vi "itc4000.vi"(9 "Temperatura":dbl min=-10.00001 max=69.99999, 10 "Corriente":dbl min=0.0 max=0.001 step=1e-05) -> (0 "Temperatura sal":dbl, 1 "Corriente sal":dbl, 2 "Power (0)":dbl)   [LabVIEW 2016]
panel:
  out "error out":errorcluster
  in  "Error In":errorcluster
  out "TEC Current":dbl
  out "TEC Voltage":dbl
  out "TEC Power":dbl
  in  "stop":bool
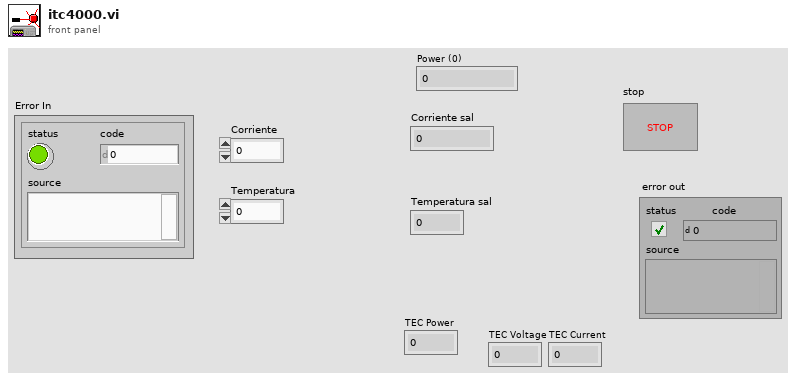
[diagram p1: front panel]
types:
  T1 = enum16{"inicio", "configurarGUI", "VALORESDEFAULT", "valordef2", "limites", "delay", "medir", "cerrar"}
  T2 = enum8{"Enabled", "Disabled", "Disabled and Grayed Out"}
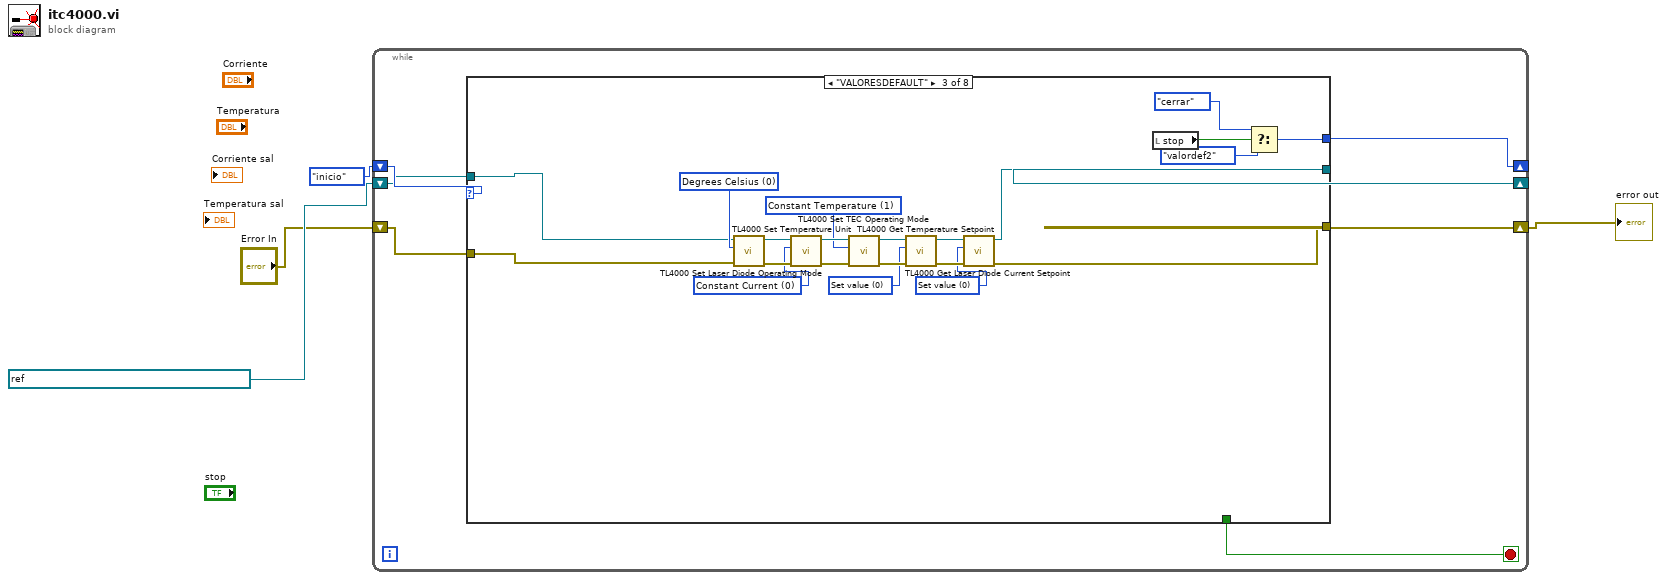
[diagram p0: block diagram]
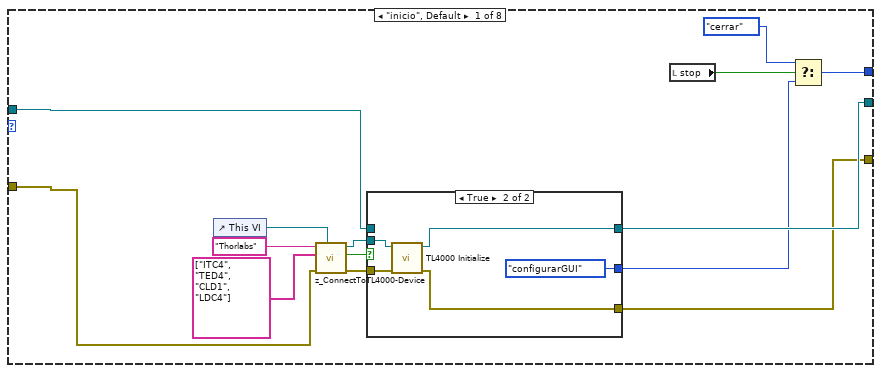
[diagram p2: hidden frame]
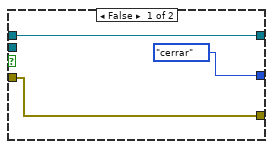
[diagram p3: hidden frame]
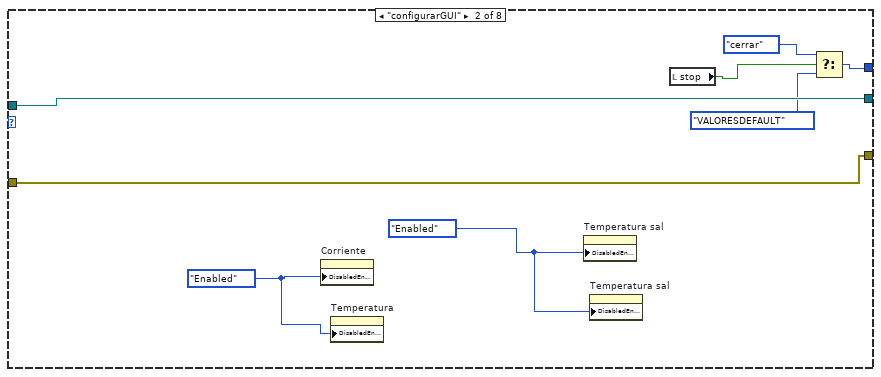
[diagram p4: hidden frame]
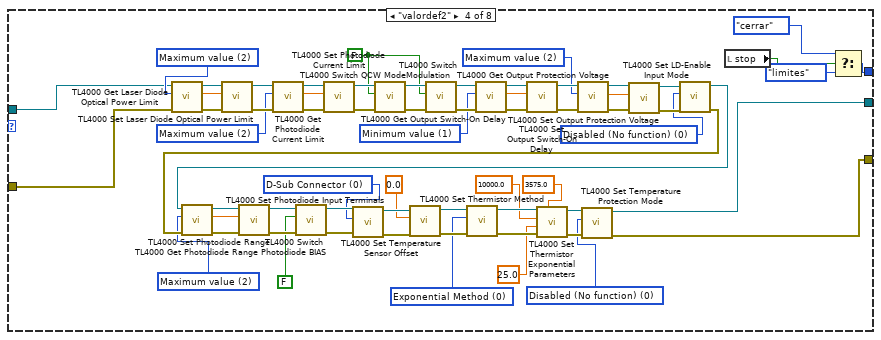
[diagram p5: hidden frame]
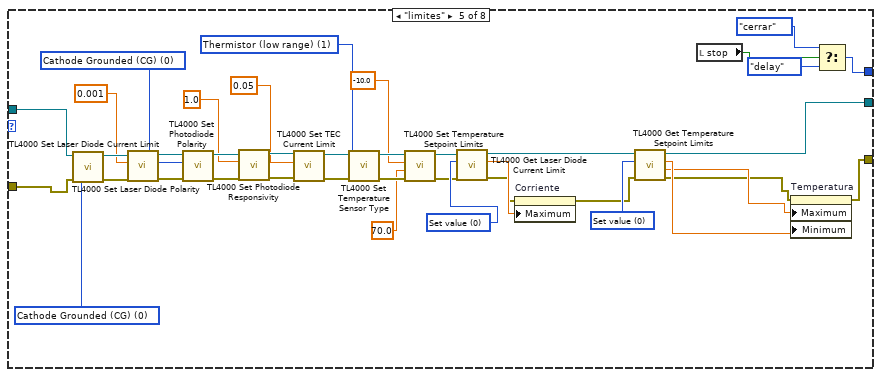
[diagram p6: hidden frame]
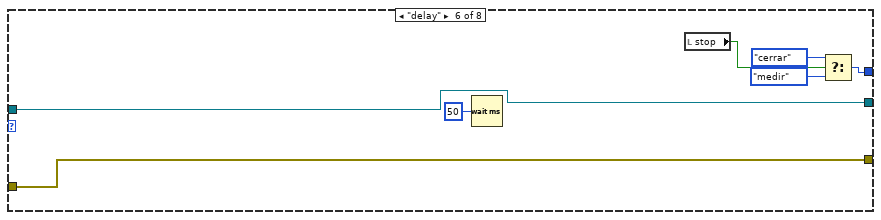
[diagram p7: hidden frame]
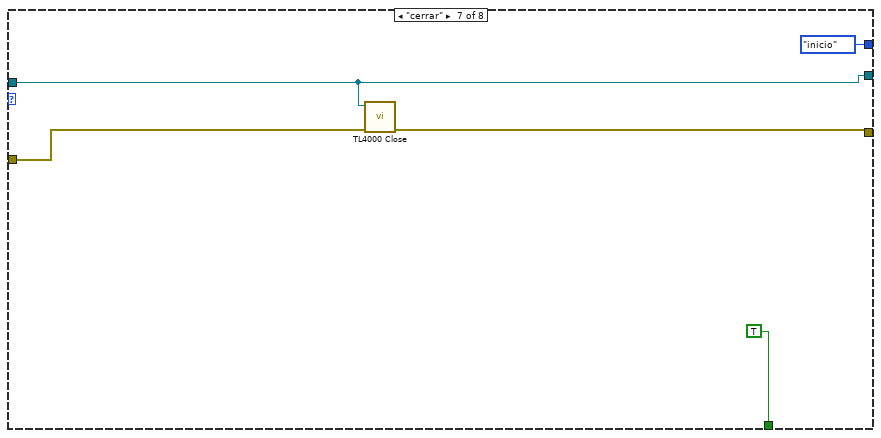
[diagram p8: hidden frame]
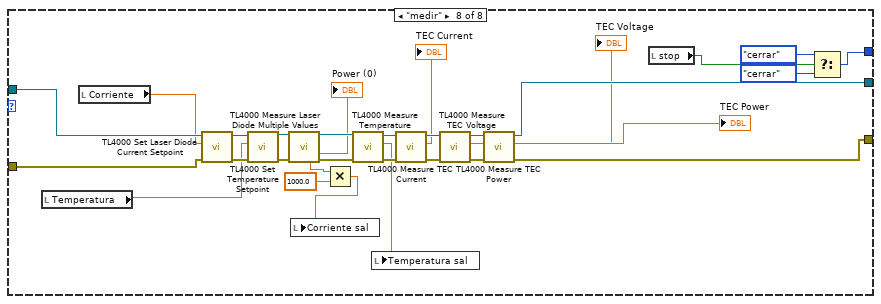
[diagram p9: hidden frame]
diagram:
  n1 = while {
    shift-right: [w6] -> _
    shift-left: T1."inicio" -> [w11]
    shift-right: [w10] -> _
    shift-left: refnum<visa-resource-name> "USB0::0x1313::0x804A::M00534841::INSTR" ("resource name") -> [w8]
    shift-right: [w9] -> w1
    shift-left: "Error In" -> [w7]
    stop <- w5 stop-if-true
    n2 = case shown="\"VALORESDEFAULT\"" w11 {
      tunnel: [w16 w41 w49 w70 w161 w171 w177 w191] -> w10
      tunnel: [w13 w40 w48 w69 w155 w170 w175 w190] -> w9
      tunnel: w8 -> [w15 w41 w47 w68 w135 w171 w177 w193]
      tunnel: w7 -> [w14 w40 w46 w67 w136 w170 w176 w192]
      tunnel: [w24 w34 w42 w64 w151 w168 T1."inicio" ("f") w179] -> w6
      tunnel: [_ _ _ _ _ _ TRUE _] -> w5
      frame "inicio", Default {
        n3 = control-ref of="This VI"() -> (w21:refnum<vi>)
        n4 = call <instrlib>:"z_ConnectToTL4000-Device.vi"("VI reference"=w21, "error in"=w14, "Models"=string[] ["ITC4", "TED4", "CLD1", "LDC4"], "Manufacturer"="Thorlabs") -> ("error out"=w18:errorcluster, "FoundUSB"=w20:bool, "USB Ref"=w19:refnum<visa-resource-name>)  [unwired: 5 in]
        n5 = case shown="True" w20 {
          tunnel: w19 -> [_ w31]
          tunnel: w18 -> [w27 w33]
          tunnel: [T1."cerrar" T1."configurarGUI"] -> w12
          tunnel: [w27 w32] -> w13
          tunnel: [w28 w30] -> w16
          tunnel: w15 -> [w28 _]
          frame False {
          }
          frame True {
            n6 = call <instrlib>:"TL4000 Initialize.vi"("error in (no error)"=w33, "resource name"=w31) -> ("error out"=w32:errorcluster, "instrument handle out"=w30:refnum<visa-resource-name>)  [unwired: 8 in]
          }
        }
        n7 = local read "stop"() -> (w25:bool)
        n8 = Select(t=T1."cerrar", s=w25, f=w12) -> (s? t:f=w24:T1)
      }
      frame "configurarGUI" {
        w38 = T2."Enabled" ("Disabled")
        w39 = T2."Enabled" ("Disabled")
        n9 = property on="Corriente" class="DigNum (strict)"("DisabledEnum"=w39) -> ()  [unwired: 2 in, 2 out]
        n10 = property on="Temperatura" class="DigNum (strict)"("DisabledEnum"=w39) -> ()  [unwired: 2 in, 2 out]
        n11 = property on="Temperatura sal" class="DigNum (strict)"("DisabledEnum"=w38) -> ()  [unwired: 2 in, 2 out]
        n12 = property on="Temperatura sal" class="DigNum (strict)"("DisabledEnum"=w38) -> ()  [unwired: 2 in, 2 out]
        n13 = local read "stop"() -> (w36:bool)
        n14 = Select(t=T1."cerrar", s=w36, f=T1."VALORESDEFAULT") -> (s? t:f=w34:T1)
      }
      frame "VALORESDEFAULT" {
        w50 = i16 0 items=["Set value", "Minimum value", "Maximum value"] ("Attribute (Set value)")
        w51 = i16 0 items=["Set value", "Minimum value", "Maximum value"] ("Attribute (Set value)")
        w52 = i16 1 items=["Constant Temperature"=1, "Current Source"=0] ("TEC Operating Mode (Constant Temperature)")
        w53 = i16 0 items=["Constant Current", "Constant Power"] ("Laser Diode Operating Mode (Constant Current)")
        w54 = i16 0 items=["Degrees Celsius", "Kelvin", "Degrees Fahrenheit"] ("Temperature Unit (Degrees Celsius)")
        n15 = call <instrlib>:"TL4000 Set Temperature Unit.vi"("error in (no error)"=w46, "Temperature Unit (Degrees Celsius)"=w54, "instrument handle"=w47) -> ("error out"=w62:errorcluster, "instrument handle out"=w58:refnum<visa-resource-name>)  [unwired: 7 in]
        n16 = call <instrlib>:"TL4000 Set Laser Diode Operating Mode.vi"("error in (no error)"=w62, "Laser Diode Operating Mode (Constant Current)"=w53, "instrument handle"=w58) -> ("error out"=w61:errorcluster, "instrument handle out"=w57:refnum<visa-resource-name>)  [unwired: 7 in]
        n17 = call <instrlib>:"TL4000 Set TEC Operating Mode.vi"("error in (no error)"=w61, "TEC Operating Mode (Constant Temperature)"=w52, "instrument handle"=w57) -> ("error out"=w60:errorcluster, "instrument handle out"=w56:refnum<visa-resource-name>)  [unwired: 7 in]
        n18 = call <instrlib>:"TL4000 Get Laser Diode Current Setpoint.vi"("error in (no error)"=w60, "Attribute (Set value)"=w51, "instrument handle"=w56) -> ("error out"=w59:errorcluster, "instrument handle out"=w55:refnum<visa-resource-name>)  [unwired: 6 in, 1 out]
        n19 = call <instrlib>:"TL4000 Get Temperature Setpoint.vi"("error in (no error)"=w59, "Attribute (Set value)"=w50, "instrument handle"=w55) -> ("error out"=w48:errorcluster, "instrument handle out"=w49:refnum<visa-resource-name>)  [unwired: 6 in, 1 out]
        n20 = local read "stop"() -> (w44:bool)
        n21 = Select(t=T1."cerrar", s=w44, f=T1."valordef2") -> (s? t:f=w42:T1)
      }
      frame "valordef2" {
        w71 = i16 0 items=["Disabled (No function)", "Output Enable", "Output Protection"] ("Mode (Disabled (No function))")
        w72 = i16 0 items=["Exponential Method", "Method from Steinhart-Hart"] ("Method (Exponential Method)")
        w74 = i16 0 items=["D-Sub Connector", "Rear Panel BNC"] ("Terminals (D-Sub Connector)")
        w76 = i16 2 items=["Set value", "Minimum value", "Maximum value"] ("Attribute (Set value)")
        w78 = i16 0 items=["Disabled (No function)", "Output Enable", "Output Protection"] ("Mode (Disabled (No function))")
        w80 = i16 2 items=["Set value", "Minimum value", "Maximum value", "Default value"] ("Attribute (Set value)")
        w82 = i16 1 items=["Set value", "Minimum value", "Maximum value", "Default value"] ("Attribute (Set value)")
        w83 = FALSE ("QCW Mode (Off)")
        w85 = i16 2 items=["Set value", "Minimum value", "Maximum value"] ("Attribute (Set value)")
        w87 = i16 2 items=["Set value", "Minimum value", "Maximum value"] ("Attribute (Set value)")
        n22 = call <instrlib>:"TL4000 Get Laser Diode Optical Power Limit.vi"("error in (no error)"=w67, "Attribute (Set value)"=w87, "instrument handle"=w68) -> ("error out"=w125:errorcluster, "Optical Power Limit"=w86:dbl, "instrument handle out"=w126:refnum<visa-resource-name>)  [unwired: 6 in]
        n23 = call <instrlib>:"TL4000 Set Laser Diode Optical Power Limit.vi"("error in (no error)"=w125, "Optical Power Limit (0.0)"=w86, "instrument handle"=w126) -> ("error out"=w123:errorcluster, "instrument handle out"=w124:refnum<visa-resource-name>)  [unwired: 7 in]
        n24 = call <instrlib>:"TL4000 Get Photodiode Current Limit.vi"("error in (no error)"=w123, "Attribute (Set value)"=w85, "instrument handle"=w124) -> ("error out"=w121:errorcluster, "Photodiode Current Limit"=w84:dbl, "instrument handle out"=w122:refnum<visa-resource-name>)  [unwired: 6 in]
        n25 = call <instrlib>:"TL4000 Set Photodiode Current Limit.vi"("error in (no error)"=w121, "Photodiode Current Limit (0.0)"=w84, "instrument handle"=w122) -> ("error out"=w119:errorcluster, "instrument handle out"=w120:refnum<visa-resource-name>)  [unwired: 7 in]
        n26 = call <instrlib>:"TL4000 Switch QCW Mode.vi"("error in (no error)"=w119, "QCW Mode (Off)"=w83, "instrument handle"=w120) -> ("error out"=w117:errorcluster, "instrument handle out"=w118:refnum<visa-resource-name>)  [unwired: 7 in]
        n27 = call <instrlib>:"TL4000 Switch Modulation.vi"("error in (no error)"=w117, "Modulation State (Off)"=w83, "instrument handle"=w118) -> ("error out"=w115:errorcluster, "instrument handle out"=w116:refnum<visa-resource-name>)  [unwired: 7 in]
        n28 = call <instrlib>:"TL4000 Get Output Switch-On Delay.vi"("error in (no error)"=w115, "Attribute (Set value)"=w82, "instrument handle"=w116) -> ("error out"=w113:errorcluster, "Delay"=w81:dbl, "instrument handle out"=w114:refnum<visa-resource-name>)  [unwired: 6 in]
        n29 = call <instrlib>:"TL4000 Set Output Switch-On Delay.vi"("error in (no error)"=w113, "Delay (1.0)"=w81, "instrument handle"=w114) -> ("error out"=w111:errorcluster, "instrument handle out"=w112:refnum<visa-resource-name>)  [unwired: 7 in]
        n30 = call <instrlib>:"TL4000 Get Output Protection Voltage.vi"("error in (no error)"=w111, "Attribute (Set value)"=w80, "instrument handle"=w112) -> ("error out"=w109:errorcluster, "Voltage"=w79:dbl, "instrument handle out"=w110:refnum<visa-resource-name>)  [unwired: 6 in]
        n31 = call <instrlib>:"TL4000 Set Output Protection Voltage.vi"("error in (no error)"=w109, "Voltage (5.0)"=w79, "instrument handle"=w110) -> ("error out"=w108:errorcluster, "instrument handle out"=w107:refnum<visa-resource-name>)  [unwired: 7 in]
        n32 = call <instrlib>:"TL4000 Set LD-Enable Input Mode.vi"("error in (no error)"=w108, "Mode (Disabled (No function))"=w78, "instrument handle"=w107) -> ("error out"=w105:errorcluster, "instrument handle out"=w106:refnum<visa-resource-name>)  [unwired: 7 in]
        n33 = call <instrlib>:"TL4000 Get Photodiode Range.vi"("error in (no error)"=w105, "Attribute (Set value)"=w76, "instrument handle"=w106) -> ("error out"=w103:errorcluster, "Range"=w77:dbl, "instrument handle out"=w104:refnum<visa-resource-name>)  [unwired: 6 in]
        n34 = call <instrlib>:"TL4000 Set Photodiode Range.vi"("error in (no error)"=w103, "Range (0.001)"=w77, "instrument handle"=w104) -> ("error out"=w101:errorcluster, "instrument handle out"=w102:refnum<visa-resource-name>)  [unwired: 7 in]
        n35 = call <instrlib>:"TL4000 Switch Photodiode BIAS.vi"("error in (no error)"=w101, "BIAS State (Off)"=FALSE, "instrument handle"=w102) -> ("error out"=w99:errorcluster, "instrument handle out"=w100:refnum<visa-resource-name>)  [unwired: 7 in]
        n36 = call <instrlib>:"TL4000 Set Photodiode Input Terminals.vi"("error in (no error)"=w99, "Terminals (D-Sub Connector)"=w74, "instrument handle"=w100) -> ("error out"=w97:errorcluster, "instrument handle out"=w98:refnum<visa-resource-name>)  [unwired: 7 in]
        n37 = call <instrlib>:"TL4000 Set Temperature Sensor Offset.vi"("error in (no error)"=w97, "Temperature Offset (0.0)"=0.0, "instrument handle"=w98) -> ("error out"=w95:errorcluster, "instrument handle out"=w96:refnum<visa-resource-name>)  [unwired: 7 in]
        n38 = call <instrlib>:"TL4000 Set Thermistor Method.vi"("error in (no error)"=w95, "Method (Exponential Method)"=w72, "instrument handle"=w96) -> ("error out"=w91:errorcluster, "instrument handle out"=w92:refnum<visa-resource-name>)  [unwired: 7 in]
        n39 = call <instrlib>:"TL4000 Set Thermistor Exponential Parameters.vi"("Beta value (3575.0)"=3575.0, "error in (no error)"=w91, "T0 value (25.0)"=25.0, "R0 value (10.0E3)"=10000.0, "instrument handle"=w92) -> ("error out"=w93:errorcluster, "instrument handle out"=w94:refnum<visa-resource-name>)  [unwired: 5 in]
        n40 = call <instrlib>:"TL4000 Set Temperature Protection Mode.vi"("error in (no error)"=w93, "Mode (Disabled (No function))"=w71, "instrument handle"=w94) -> ("error out"=w69:errorcluster, "instrument handle out"=w70:refnum<visa-resource-name>)  [unwired: 7 in]
        n41 = local read "stop"() -> (w65:bool)
        n42 = Select(t=T1."cerrar", s=w65, f=T1."limites") -> (s? t:f=w64:T1)
      }
      frame "limites" {
        w129 = i16 1 items=["AD590", "Thermistor (low range)", "Thermistor (high range)", "PT100", "PT1000", "LM35", "LM335"] ("Sensor (AD590)")
        w132 = i16 0 items=["Cathode Grounded (CG)", "Anode Grounded (AG)"] ("Polarity (Cathode Grounded (CG))")
        w134 = i16 0 items=["Cathode Grounded (CG)", "Anode Grounded (AG)"] ("Polarity (Cathode Grounded (CG))")
        w165 = i16 0 items=["Set value", "Minimum value", "Maximum value"] ("Attribute (Set value)")
        w164 = i16 0 items=["Set value", "Minimum value", "Maximum value"] ("Attribute (Set value)")
        n43 = call <instrlib>:"TL4000 Set Laser Diode Polarity.vi"("error in (no error)"=w136, "Polarity (Cathode Grounded (CG))"=w134, "instrument handle"=w135) -> ("error out"=w149:errorcluster, "instrument handle out"=w150:refnum<visa-resource-name>)  [unwired: 7 in]
        n44 = call <instrlib>:"TL4000 Set Laser Diode Current Limit.vi"("error in (no error)"=w149, "Laser Diode Current Limit (0.0)"=0.001, "instrument handle"=w150) -> ("error out"=w147:errorcluster, "instrument handle out"=w148:refnum<visa-resource-name>)  [unwired: 7 in]
        n45 = call <instrlib>:"TL4000 Set Photodiode Polarity.vi"("error in (no error)"=w147, "Polarity (Cathode Grounded (CG))"=w132, "instrument handle"=w148) -> ("error out"=w145:errorcluster, "instrument handle out"=w146:refnum<visa-resource-name>)  [unwired: 7 in]
        n46 = call <instrlib>:"TL4000 Set Photodiode Responsivity.vi"("error in (no error)"=w145, "Responsivity (1.0)"=1.0, "instrument handle"=w146) -> ("error out"=w143:errorcluster, "instrument handle out"=w144:refnum<visa-resource-name>)  [unwired: 7 in]
        n47 = call <instrlib>:"TL4000 Set TEC Current Limit.vi"("error in (no error)"=w143, "TEC Current Limit (1.0)"=0.05, "instrument handle"=w144) -> ("error out"=w141:errorcluster, "instrument handle out"=w142:refnum<visa-resource-name>)  [unwired: 7 in]
        n48 = call <instrlib>:"TL4000 Set Temperature Sensor Type.vi"("error in (no error)"=w141, "Sensor (AD590)"=w129, "instrument handle"=w142) -> ("error out"=w139:errorcluster, "instrument handle out"=w140:refnum<visa-resource-name>)  [unwired: 7 in]
        n49 = call <instrlib>:"TL4000 Set Temperature Setpoint Limits.vi"("error in (no error)"=w139, "Setpoint High Limit (50.0)"=70.0, "Setpoint Low Limit (0.0)"=-10.0, "instrument handle"=w140) -> ("error out"=w137:errorcluster, "instrument handle out"=w138:refnum<visa-resource-name>)  [unwired: 6 in]
        n50 = call <instrlib>:"TL4000 Get Laser Diode Current Limit.vi"("error in (no error)"=w137, "Attribute (Set value)"=w164, "instrument handle"=w138) -> ("error out"=w157:errorcluster, "Laser Diode Current Limit"=w162:dbl, "instrument handle out"=w163:refnum<visa-resource-name>)  [unwired: 6 in]
        n51 = property on="Corriente" class="DigNum (strict)"(error in=w157, "Maximum"=w162) -> (error out=w156:errorcluster)  [unwired: 1 in, 1 out]
        n52 = call <instrlib>:"TL4000 Get Temperature Setpoint Limits.vi"("error in (no error)"=w156, "Attribute (Set value)"=w165, "instrument handle"=w163) -> ("error out"=w158:errorcluster, "Setpoint High Limit"=w159:dbl, "Setpoint Low Limit"=w160:dbl, "instrument handle out"=w161:refnum<visa-resource-name>)  [unwired: 5 in]
        n53 = local read "stop"() -> (w153:bool)
        n54 = property on="Temperatura" class="DigNum (strict)"(error in=w158, "Maximum"=w159, "Minimum"=w160) -> (error out=w155:errorcluster)  [unwired: 1 in, 1 out]
        n55 = Select(t=T1."cerrar", s=w153, f=T1."delay") -> (s? t:f=w151:T1)
      }
      frame "delay" {
        n56 = Wait (ms)(milliseconds to wait=u32 50) -> ()  [unwired: 1 out]
        n57 = local read "stop"() -> (w167:bool)
        n58 = Select(t=T1."cerrar", s=w167, f=T1."medir") -> (s? t:f=w168:T1)
      }
      frame "cerrar" {
        n59 = call <instrlib>:"TL4000 Close.vi"("error in (no error)"=w176, "instrument handle"=w177) -> ("error out"=w175:errorcluster)  [unwired: 9 in]
      }
      frame "medir" {
        n60 = local read "Temperatura"() -> (w183:dbl)
        n61 = local read "Corriente"() -> (w178:dbl)
        n62 = call <instrlib>:"TL4000 Set Laser Diode Current Setpoint.vi"("error in (no error)"=w192, "Laser Diode Current Setpoint (0.0)"=w178, "instrument handle"=w193) -> ("error out"=w194:errorcluster, "instrument handle out"=w195:refnum<visa-resource-name>)  [unwired: 7 in]
        n63 = call <instrlib>:"TL4000 Set Temperature Setpoint.vi"("error in (no error)"=w194, "Temperature Setpoint (25.0)"=w183, "instrument handle"=w195) -> ("error out"=w202:errorcluster, "instrument handle out"=w203:refnum<visa-resource-name>)  [unwired: 7 in]
        n64 = call <instrlib>:"TL4000 Measure Laser Diode Multiple Values.vi"("instrument handle"=w203, "error in (no error)"=w202) -> ("instrument handle out"=w200:refnum<visa-resource-name>, "Power (0)"=→"Power (0)":dbl, "Photodiode Current (0)"=w197:dbl, "error out"=w201:errorcluster)  [unwired: 5 in, 5 out]
        n65 = Multiply(x=w197, y=1000.0) -> (x*y=w184:dbl)
        n66 = local write "Corriente sal"(w184) -> ()
        n67 = call <instrlib>:"TL4000 Measure Temperature.vi"("error in (no error)"=w201, "instrument handle"=w200) -> ("error out"=w198:errorcluster, "Temperature"=w185:dbl, "instrument handle out"=w199:refnum<visa-resource-name>)  [unwired: 7 in]
        n68 = local write "Temperatura sal"(w185) -> ()
        n69 = call <instrlib>:"TL4000 Measure TEC Current.vi"("error in (no error)"=w198, "instrument handle"=w199) -> ("error out"=w206:errorcluster, "TEC Current"=→"TEC Current":dbl, "instrument handle out"=w207:refnum<visa-resource-name>)  [unwired: 7 in]
        n70 = call <instrlib>:"TL4000 Measure TEC Voltage.vi"("error in (no error)"=w206, "instrument handle"=w207) -> ("error out"=w204:errorcluster, "TEC Voltage"=→"TEC Voltage":dbl, "instrument handle out"=w205:refnum<visa-resource-name>)  [unwired: 7 in]
        n71 = call <instrlib>:"TL4000 Measure TEC Power.vi"("error in (no error)"=w204, "instrument handle"=w205) -> ("error out"=w190:errorcluster, "TEC Power"=→"TEC Power":dbl, "instrument handle out"=w191:refnum<visa-resource-name>)  [unwired: 7 in]
        n72 = local read "stop"() -> (w181:bool)
        n73 = Select(t=T1."cerrar", s=w181, f=T1."cerrar") -> (s? t:f=w179:T1)
      }
    }
  }
  "error out" <- w1
